vi "Set error - SubVI.vi"(0 "code":i32, 2 "Additional information":string, 5 "error in":errorcluster) -> (8 "error out":errorcluster)   [LabVIEW 2014]
uses:
  Lambda Globals.vi
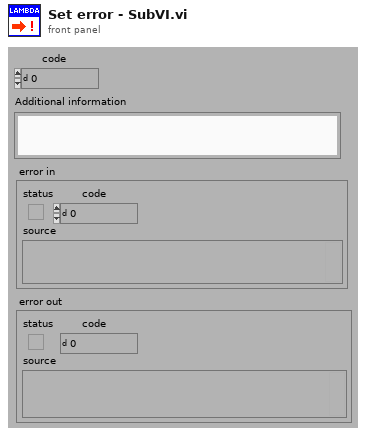
[diagram p1: front panel]
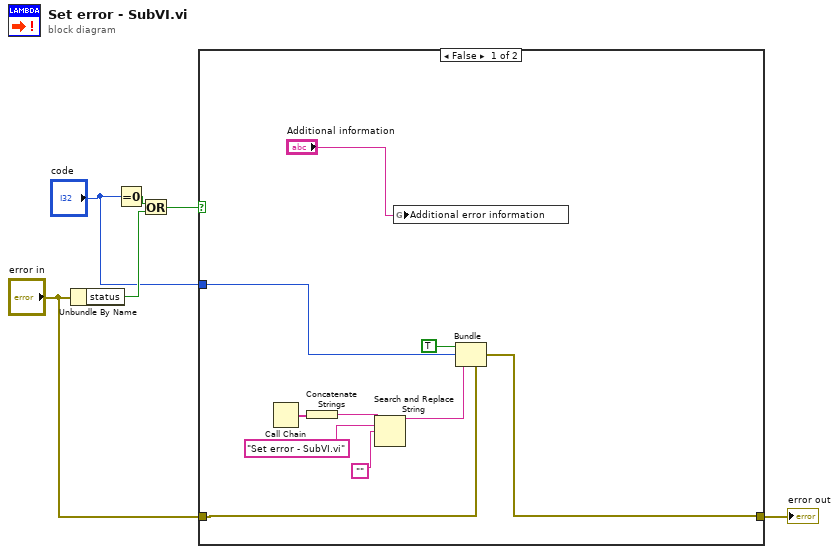
[diagram p0: block diagram]
diagram:
  n1 = Unbundle By Name("error in") -> ("status"=w3:bool)
  n2 = Equal To 0?(x="code") -> (x = 0?=w4:bool)
  n3 = Or(x=w4, y=w3) -> (x .or. y?=w2:bool)
  n4 = case shown="False" w2 {
    tunnel: [w11 w17] -> w6
    tunnel: "error in" -> [w12 w17]
    tunnel: "code" -> [w7 _]
    frame False {
      n5 = Call Chain() -> (call chain=w14:string[])
      n6 = Concatenate Strings(w14) -> (w13:string)
      n7 = Search and Replace String(input string=w13, search string="Set error - SubVI.vi", replace string="") -> (result string=w10:string)  [unwired: 1 in, 7 out]
      n8 = global write "Lambda Globals.vi" "Additional error information"("Additional information") -> ()
      n9 = Bundle(cluster=w12, "status"=TRUE, "code"=w7, "source"=w10) -> (w11:errorcluster)
    }
    frame True {
    }
  }
  "error out" <- w6
